vi "MainVI.vi"() -> ()   [LabVIEW 2022 SP3]
uses:
  <vilib>/Simulation/Scripting/Companion Diagram/SimConfigNode/SimParams.ctl
  <vilib>/Simulation/Scripting/Companion Diagram/SimConfigNode/_simSolvers.ctl
  <vilib>/Simulation/Implementation/Shared/SIMSCR Execution Mode.ctl
  <vilib>/Simulation/Param Hierarchy/Typedefs/SIMPH Param Control Actions.ctl
  <vilib>/OPCUA/controls/NodeId.ctl
  <vilib>/OPCUA/controls/Write Status.ctl
  <vilib>/Simulation/Implementation/Shared/NILVSim_ParamChanged.vi
  <vilib>/Simulation/Implementation/Shared/NILVSIM_BeginStep.vi
  <vilib>/Simulation/Implementation/Shared/NILVSim_Manager.vi
  <vilib>/Utility/error.llb/Clear Errors.vi
  <vilib>/Simulation/Implementation/Shared/NILVSim_FinalizeModel.vi
  <vilib>/Simulation/Implementation/Shared/SIM Unbundle Sim Info.vi
  <vilib>/Simulation/Implementation/Shared/NILVSim_Initialize.vi
  <vilib>/Simulation/Utility/Implementation/NILVSim Get Time and IsAcceptedStep.vi
  <vilib>/Simulation/Implementation/Shared/SIMSH Read Queue.vi
  <vilib>/Simulation/Implementation/Shared/NILVSim_GetModelError.vi
  <vilib>/Simulation/Implementation/Shared/SIM Bundle Sim Info.vi
  <vilib>/OPCUA/client/Multiple Write Double.vi
  <vilib>/Simulation/Implementation/XNodeFramework/SimXNode/SimX.xnode
  SubVI/Mathematical Model Air Heater.vi
  <vilib>/Simulation/Scripting/Companion Diagram/SimConfigNode/SimDog.xnode
  <vilib>/Simulation/Implementation/Shared/NI_SIM_Implementation.lvlib
  <vilib>/OPCUA/NI OPC UA Client.lvlib
panel:
  out "T_env [Deg C]":dbl caption="Environment \nTemperature [Deg C]" format="%.1g"
  out "Temperature Chart":T1(graph)
  out "Control Signal [V]":dbl(slide)=1.1413304392579737 scale=0.0..5.0
  in  "Tab Control":enum32{"Process", "Controller"}(tab)=enum."Controller"
  in  "Simulation":bool=TRUE
  in  "Model Parameters":T2={"K [C/V]"=3.5, "T_delay [s]"=2.0, "T_env [Deg C]"=21.5, "T initial [Deg C]"=21.5, "T [s]"=22.0}
  in  "PI Controller":bool=TRUE caption="Controller"
  in  "Manual Control [V]":dbl(slide) scale=0.0..5.0
  in  "PI Parameters":cluster{"Kp":dbl, "Ti [s]":dbl}={"Kp"=0.8, "Ti [s]"=20.0}
  in  "Control Signal Range":cluster{"u_max":dbl, "u_min":dbl}={"u_max"=5.0, "u_min"=0.0}
  out "Name":string
  in  "Setpoint [Deg C]":dbl=30.0
  in  "Ts [s]":dbl=0.1
  in  "Stop Button":bool
  out "Temperature [Deg C]":dbl(slide)=21.64553529889341 scale=20.0..50.0
  out "Error out":errorcluster
  in  "Error in":errorcluster
  # "Control Module"
  # "Simulation"
  # "Real"
  # "PI Controller"
  # "Manual Controller"
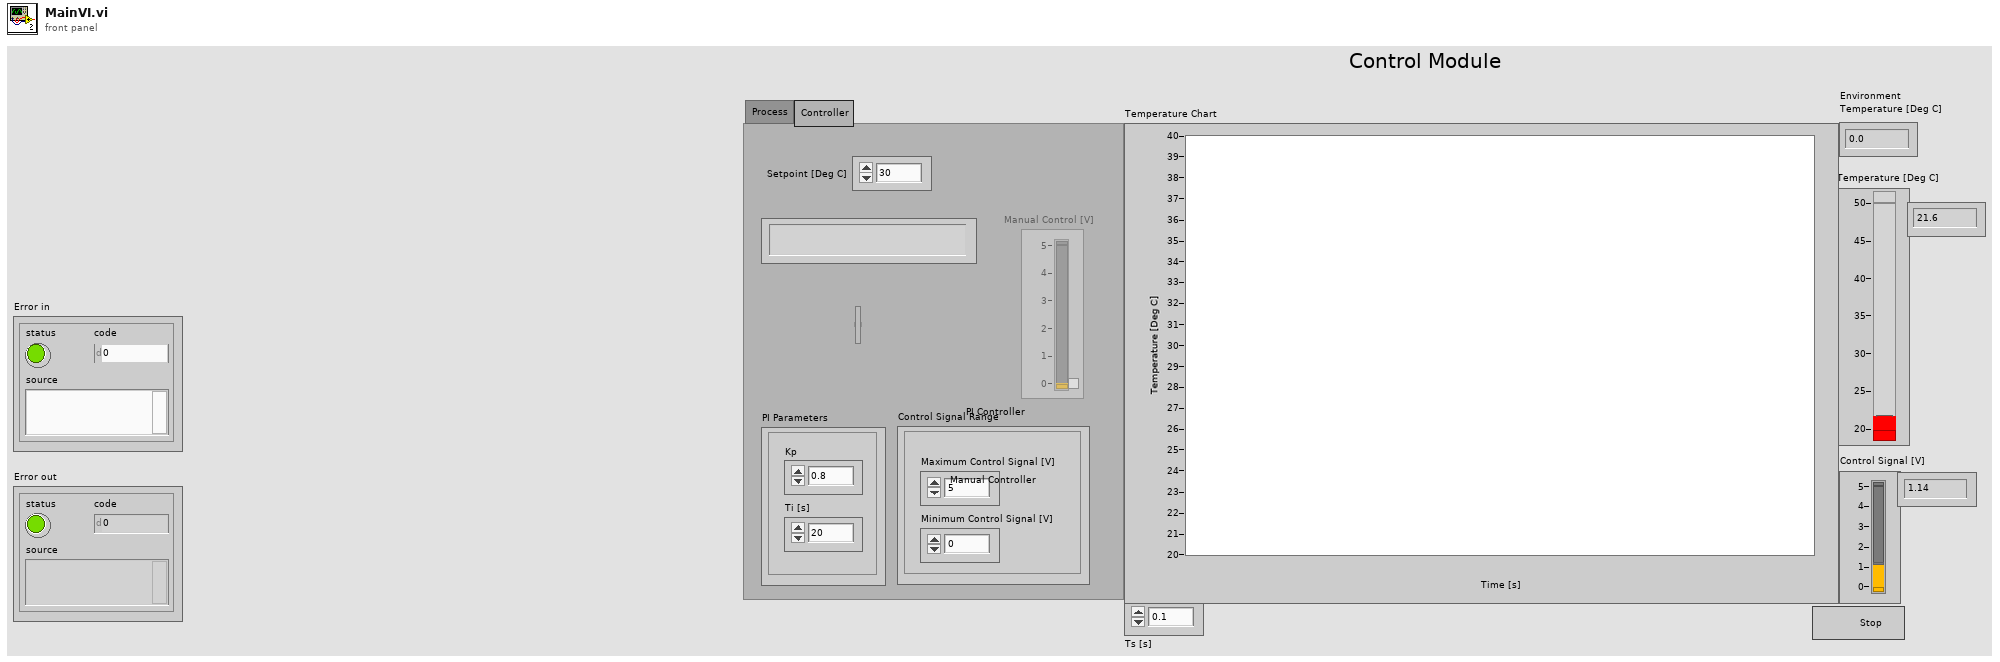
[diagram p1: front panel]
types:
  T1 = cluster{"T_out [deg C]":dbl, "Setpoint [Deg C]":dbl}
  T2 = cluster{"K [C/V]":dbl, "T_delay [s]":dbl, "T_env [Deg C]":dbl, "T initial [Deg C]":dbl, "T [s]":dbl}
  T3 = cluster{"T_out [deg C]":dbl, "Setpoint [Deg C]":dbl}[]
  T4 = enum8{"Enabled", "Disabled", "Disabled and Grayed Out"}
  T5 = enum16{"Simulate to Completion", "Single Time-Step Simulation (Fixed Step Only)"}
  T6 = typedef "SIMSCR Execution Mode.ctl" = enum16{"Simulate to Completion", "Single Time-Step Simulation (Fixed Step Only)"}
  T7 = typedef "SIMPH Param Control Actions.ctl" = enum16{"get params", "set params"}
  T8 = cluster{"SIMSH Sim Time":dbl, "Unbundle By Name":cluster{"K [C/V]":dbl, "T_delay [s]":dbl, "T_env [Deg C]":dbl, "T initial [Deg C]":dbl, "T [s]":dbl}, "Model Parameters":cluster{"K [C/V]":dbl, "T_delay [s]":dbl, "T_env [Deg C]":dbl, "T initial [Deg C]":dbl, "T [s]":dbl}, "Integrator":cluster{"output":dbl}, "Devision":cluster{"Result":dbl}, "Minus":cluster{"Result":dbl}, "Transport Delay":cluster{"output":dbl}, "Summation":cluster{"Result":dbl}, "Multiplication":cluster{"Result":dbl}}
  T9 = typedef "SimParams.ctl" = cluster{"Initial Time (s)":dbl, "Final Time (s)":dbl, "Step Size (s)":dbl, "ODE Solver":T10, "Minimum Step Size (s)":dbl, "Maximum Step Size (s)":dbl, "Relative Tolerance":dbl, "Absolute Tolerance":dbl, "Software Timing":bool, "Initial Step Size (s)":dbl, "Automatic Fixed Step Size?":bool, "Automatic Discrete Step Size?":bool, "Discrete Step Size (s)":dbl, "Calculate using Time Step":bool, "Solver Wired?":bool, "Prev.Frm.Expected End":u64, "Prev.Frm.Actual End":u64, "Prev.Frm.Finished Late?":bool, "Prev.Iter.Expected End":u64, "Prev.Iter.Actual End":u64, "Prev.Iter.Finished Late?":bool, "Expected Iteration Start":u64, "Actual Iteration Start":u64, "Expected Frame Start":u64, "Actual Frame Start":u64, "Source Name":string, "Name":string, "Period":i64, "Deadline":i64, "Offset":i64, "Start":i64, "Priority":i32, "Timeout":i32, "Processor":i32, "Mode":enum32{"No Change", "Process missed periods, maintain original phase", "Discard missed periods, maintain original phase", "Process missed periods, ignore original phase", "Discard missed periods, ignore original phase"}, "Wakeup reason":enum32{"Normal", "Aborted", "Asynchronous wakeup", "Timing source error", "Timed loop error", "Timeout"}, "Error":errorcluster, "Source Type":string, "Secondary Source Type":string, "Global End Time":u64, "Global Start Time":u64, "Full Solver Reset":bool, "Execution Mode":T6, "Nan/Inf Check":bool, "Custom Solver Library":string, "Solver Is Variable":bool, "custom solver name":string, "Signal Collection Decimation":u32}
  T10 = typedef "_simSolvers.ctl" = enum16{"Runge-Kutta 1 (Euler)", "Runge-Kutta 2", "Runge-Kutta 3", "Runge-Kutta 4", "Runge-Kutta 23 (variable)", "Runge-Kutta 45 (variable)", "BDF (variable)", "Adams-Moulton (variable)", "Rosenbrock (variable)", "Discrete States Only", "SDIRK 4 (variable)", "Radau 5 (variable)", "Radau 9 (variable)", "Radau 13 (variable)", "Radau [Variable Order] (variable)", "Gear's Method (variable)", "Linearizer", "State Query", "Trim Eval", "Custom Solver"}
  T11 = typedef "NodeId.ctl" = string
  T12 = cluster{"message mode":enum16{"None", "Sign", "Sign and Encrypt"}, "security":enum16{"Basic256", "Basic128Rsa15"}}
  T13 = typedef "OPC UA Client Refnum.ctl" = refnum<k21>
  T14 = cluster{"Filter Output":dbl, "Setpoint [Deg C]":dbl}
  T15 = cluster{"Setpoint [Deg C]":dbl, "Temperature [Deg C]":dbl}
  T16 = typedef "Write Status.ctl" = u32
  T17 = cluster{"node ID":T11, "value":dbl, "timestamp (current time)":timestamp, "node status":T16}
  T18 = cluster{"node ID":T11, "value":dbl, "timestamp (current time)":timestamp, "node status":T16}[]
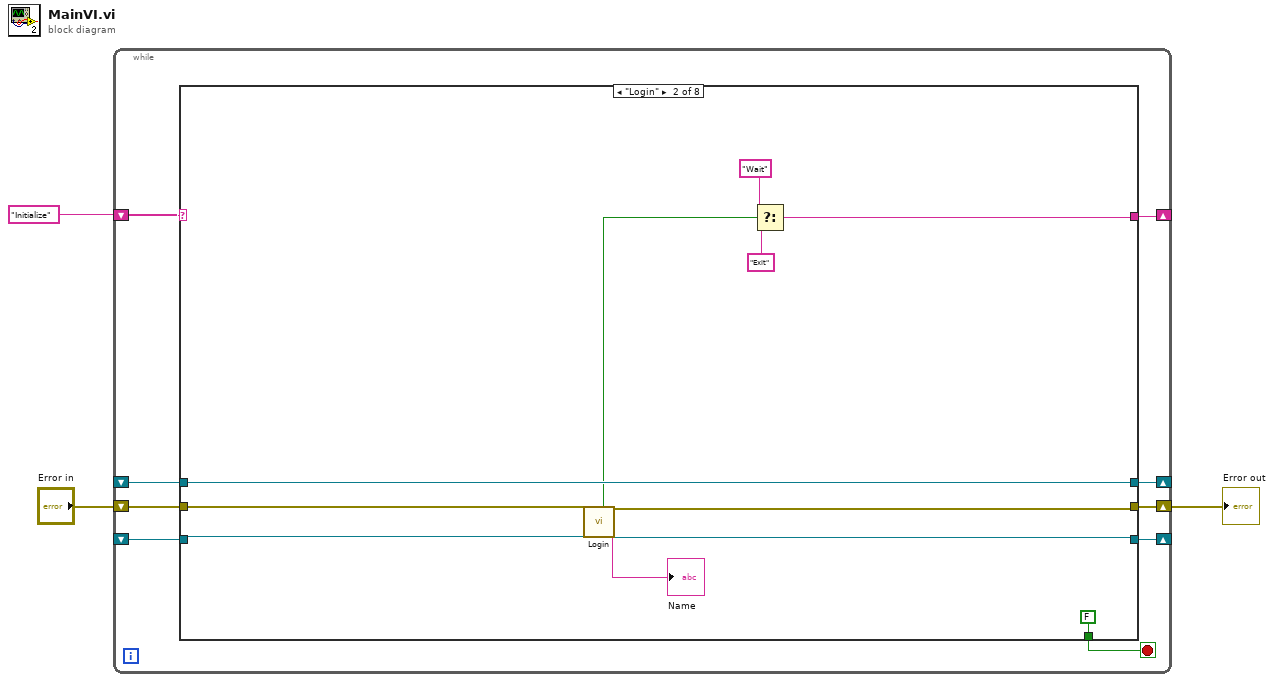
[diagram p0: block diagram]
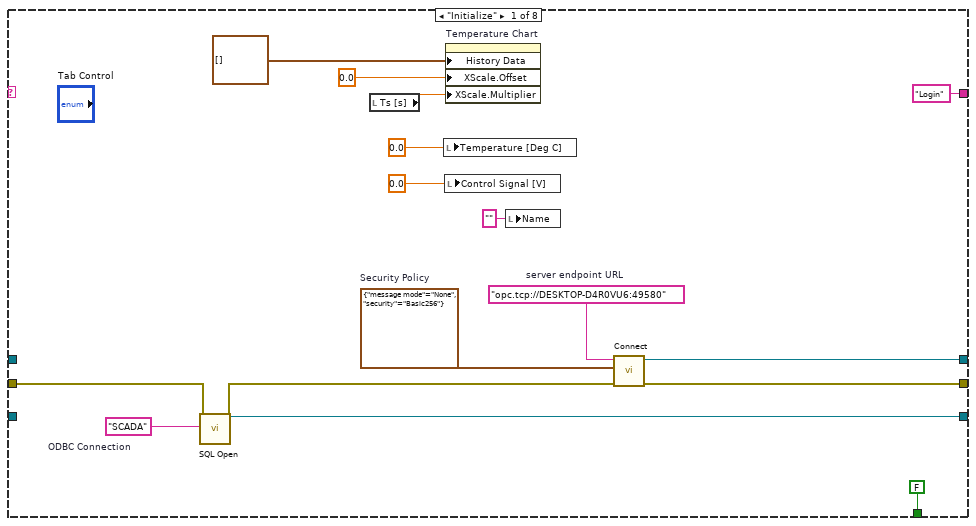
[diagram p2: hidden frame]
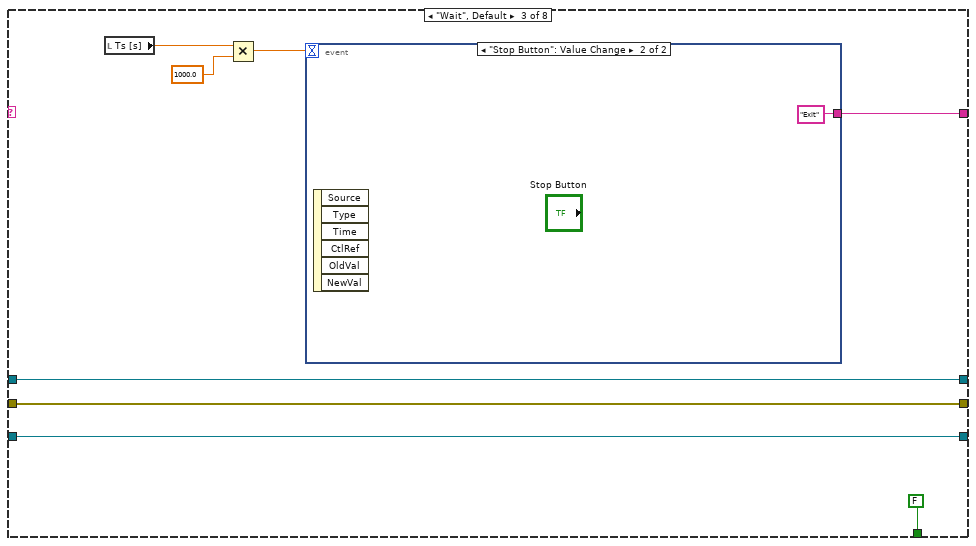
[diagram p3: hidden frame]
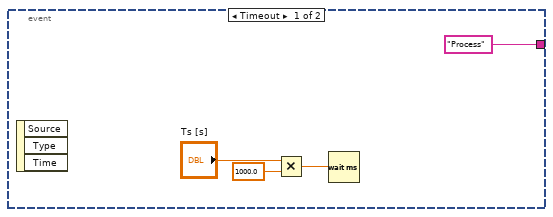
[diagram p4: hidden frame]
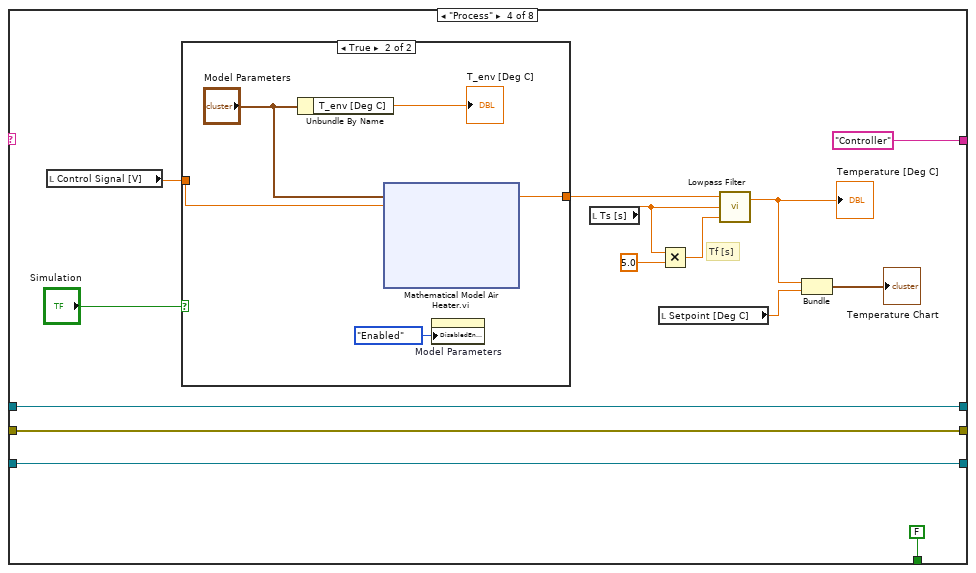
[diagram p5: hidden frame]
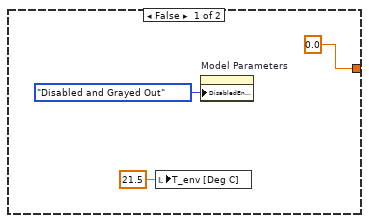
[diagram p6: hidden frame]
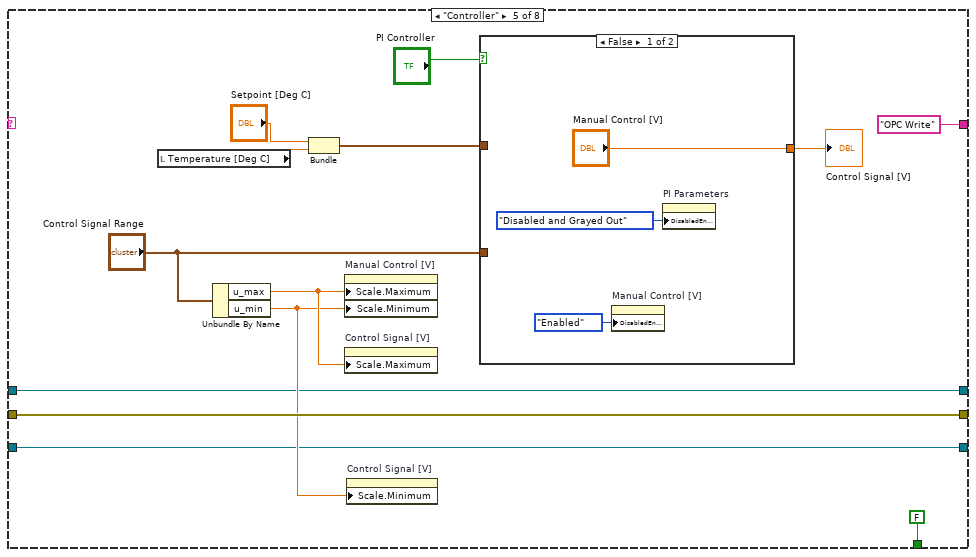
[diagram p7: hidden frame]
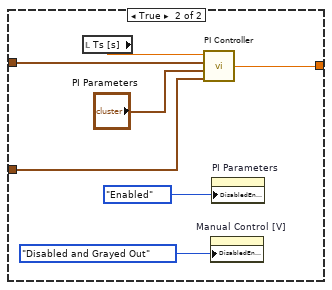
[diagram p8: hidden frame]
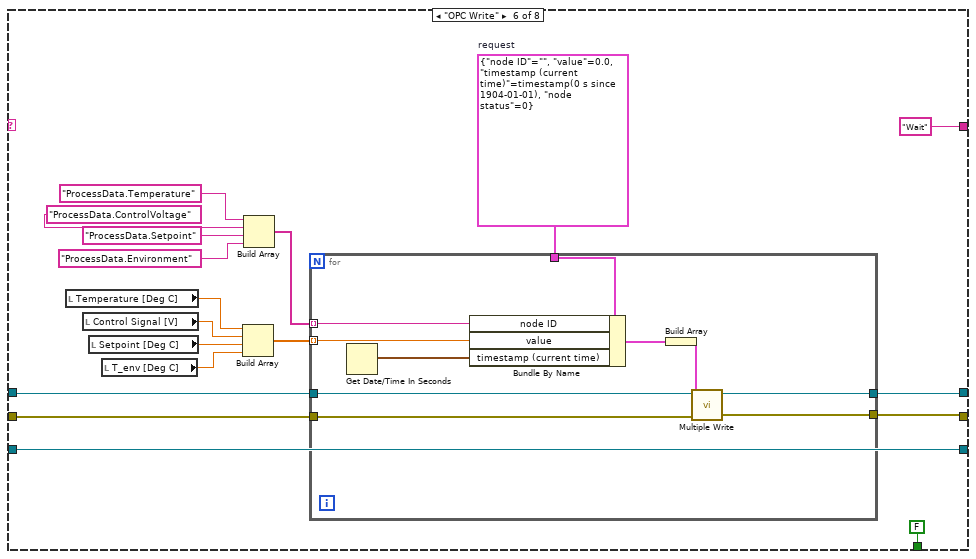
[diagram p9: hidden frame]
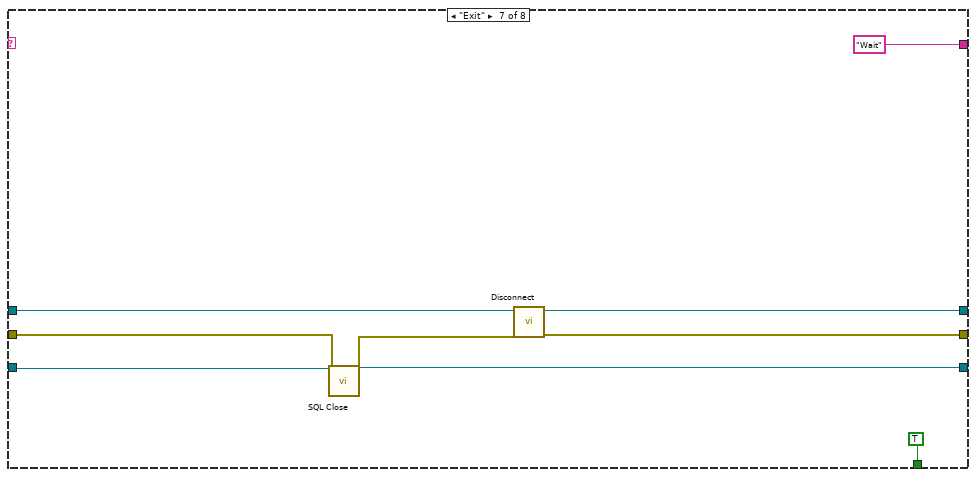
[diagram p10: hidden frame]
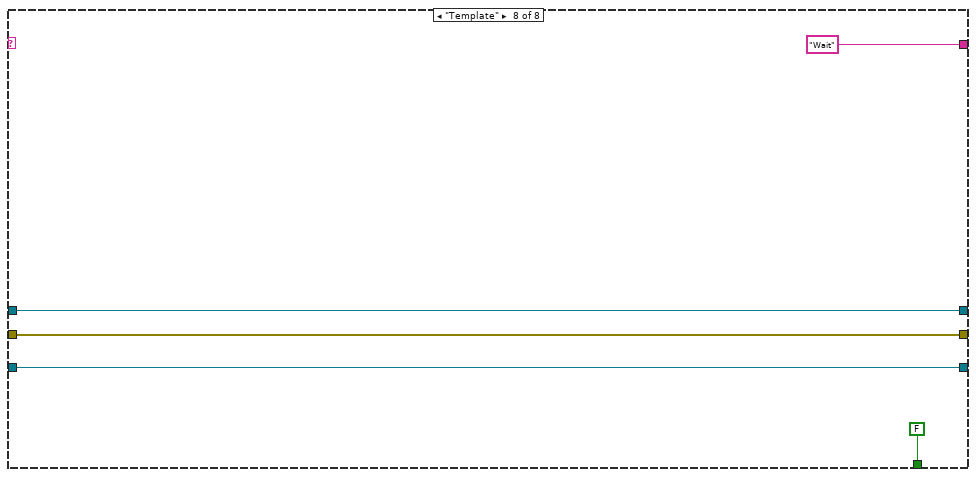
[diagram p11: hidden frame]
diagram:
  n1 = while {
    shift-right: [w11] -> _
    shift-left: "Initialize" -> [w12]
    shift-right: [w8] -> w1
    shift-left: "Error in" -> [w9]
    shift-right: [w7] -> _
    shift-left: _ -> [w6]
    shift-right: [w5] -> _
    shift-left: _ -> [w4]
    stop <- w10 stop-if-true
    n2 = case shown="\"Login\"" w12 {
      tunnel: ["Login" ("f") w34 w46 "Controller" "OPC Write" "Wait" "Wait" "Wait"] -> w11
      tunnel: [FALSE FALSE FALSE FALSE FALSE FALSE TRUE FALSE] -> w10
      tunnel: w9 -> [w17 w32 w42 w62 w333 w355 w378 w386]
      tunnel: [w21 w31 w42 w62 w333 w354 w381 w386] -> w8
      tunnel: [w19 w39 w41 w54 w327 w352 w380 w385] -> w7
      tunnel: w6 -> [_ w39 w41 w54 w327 w353 w380 w385]
      tunnel: [w15 w29 w40 w53 w326 w349 w379 w384] -> w5
      tunnel: w4 -> [_ w30 w40 w53 w326 w349 w379 w384]
      frame "Initialize" {
        w18 = "SCADA"  # ODBC Connection
        w22 = T12 {"message mode"=enum."None", "security"=enum."Basic256"}  # Security Policy
        w23 = "opc.tcp://DESKTOP-D4R0VU6:49580"  # server endpoint URL
        n3 = call <vilib>:"SQL Open.vi"("ConnectionString In"=w18, "Error in (no error)"=w17) -> ("Connection Out"=w15:refnum<k7>, "Error out"=w16:errorcluster)  [unwired: 16 in]
        n4 = local read "Ts [s]"() -> (w25:dbl)
        n5 = local write "Temperature [Deg C]"(0.0 ("Thermometer")) -> ()
        n6 = local write "Control Signal [V]"(0.0 ("Control Signal [V]")) -> ()
        n7 = property on="Temperature Chart" class="WFChart (strict)"("History Data"=T3 [], "XScale.Offset"=0.0 ("X Scale.Offset and Multiplier:Offset"), "XScale.Multiplier"=w25) -> ()  [unwired: 2 in, 2 out]
        n8 = local write "Name"("" ("Name")) -> ()
        n9 = call <vilib>:"Connect.vi"("error in (no error)"=w16, "security policy"=w22, "server endpoint URL"=w23) -> ("error out"=w21:errorcluster, "OPC UA client refnum out"=w19:T13)  [unwired: 6 in, 1 out]
      }
      frame "Login" {
        n10 = call "Login.vi"("Connection In"=w30, "error in"=w32) -> ("Not empty?"=w37:bool, "error out"=w31:errorcluster, "Connection Out"=w29:refnum<k7>, "Name"=→"Name":string)  [unwired: 2 out]
        n11 = Select(t="Wait", s=w37, f="Exit") -> (s? t:f=w34:string)
      }
      frame "Wait", Default {
        n12 = local read "Ts [s]"() -> (w45:dbl)
        n13 = Multiply(x=w45, y=1000.0) -> (x*y=w43:dbl)
        n14 = event shown="[1] \"Stop Button\": Value Change" {
          selector: _ -> [_ _]
          dyn-events: _ -> [_ _]
          timeout: w43 -> [_ _]
          tunnel: ["Process" "Exit"] -> w46
          event Timeout {
            n15 = event-data() -> ()  [unwired: 1 in, 3 out]
            n16 = Multiply(x="Ts [s]", y=1000.0) -> (x*y=w48:dbl)
            n17 = Wait (ms)(milliseconds to wait=w48) -> ()  [unwired: 1 out]
          }
          event "Stop Button": Value Change {
            n18 = event-data() -> ()  [unwired: 1 in, 6 out]
          }
        }
      }
      frame "Process" {
        # "Tf [s]"
        n19 = local read "Control Signal [V]"() -> (w63:dbl)
        n20 = case shown="True" "Simulation" {
          tunnel: [0.0 ("T_out [deg C]") w74] -> w58
          tunnel: w63 -> [_ w73]
          frame False {
            n21 = local write "T_env [Deg C]"(21.5 ("T_env [Deg C]")) -> ()
            n22 = property on="Model Parameters" class="Clust (strict)"("DisabledEnum"=T4."Disabled and Grayed Out" ("Disabled")) -> ()  [unwired: 2 in, 2 out]
          }
          frame True {
            n23 = Unbundle By Name("Model Parameters") -> ("T_env [Deg C]"=→"T_env [Deg C]":dbl)
            n24 = xnode "Mathematical Model Air Heater.vi"("Model Parameters"="Model Parameters", "u [V]"=w73) -> ("T_out [deg C]"=w74:dbl)  [unwired: 2 in, 1 out]
            n25 = property on="Model Parameters" class="Clust (strict)"("DisabledEnum"=T4."Enabled" ("Disabled")) -> ()  [unwired: 2 in, 2 out]
          }
        }
        n26 = local read "Ts [s]"() -> (w57:dbl)
        n27 = local read "Setpoint [Deg C]"() -> (w61:dbl)
        n28 = Multiply(x=w57, y=5.0) -> (x*y=w55:dbl)
        n29 = call "Lowpass Filter.vi"("Tf [s]"=w55, "Ts [s]"=w57, "Fillter input"=w58) -> ("Filter Output"=w59:dbl)  [unwired: 1 in]
        "Temperature [Deg C]" <- w59
        n30 = Bundle "Bundle"("Filter Output"=w59, "Setpoint [Deg C]"=w61) -> (→"Temperature Chart":T14)  [unwired: 1 in]
      }
      frame "Controller" {
        n31 = local read "Temperature [Deg C]"() -> (w331:dbl)
        n32 = Unbundle By Name "Unbundle By Name"("Control Signal Range") -> ("u_max"=w329:dbl, "u_min"=w328:dbl)
        n33 = Bundle("Setpoint [Deg C]"="Setpoint [Deg C]", "Temperature [Deg C]"=w331) -> (w330:T15)  [unwired: 1 in]
        n34 = property on="Manual Control [V]" class="Slide (strict)"("Scale.Maximum"=w329, "Scale.Minimum"=w328) -> ()  [unwired: 2 in, 2 out]
        n35 = property on="Control Signal [V]" class="Slide (strict)"("Scale.Maximum"=w329) -> ()  [unwired: 2 in, 2 out]
        n36 = property on="Control Signal [V]" class="Slide (strict)"("Scale.Minimum"=w328) -> ()  [unwired: 2 in, 2 out]
        n37 = case shown="False" "PI Controller" {
          tunnel: ["Manual Control [V]" w345] -> w336
          tunnel: "Control Signal Range" -> [_ w344]
          tunnel: w330 -> [_ w343]
          frame False {
            n38 = property on="Manual Control [V]" class="Slide (strict)"("DisabledEnum"=T4."Enabled" ("Disabled")) -> ()  [unwired: 2 in, 2 out]
            n39 = property on="PI Parameters" class="Clust (strict)"("DisabledEnum"=T4."Disabled and Grayed Out" ("Disabled")) -> ()  [unwired: 2 in, 2 out]
          }
          frame True {
            n40 = local read "Ts [s]"() -> (w347:dbl)
            n41 = call "PI Controller.vi"("Control Signal Range"=w344, "PI Parameters"="PI Parameters", "Process"=w343, "Ts [s]"=w347) -> ("Output"=w345:dbl)
            n42 = property on="Manual Control [V]" class="Slide (strict)"("DisabledEnum"=T4."Disabled and Grayed Out" ("Disabled")) -> ()  [unwired: 2 in, 2 out]
            n43 = property on="PI Parameters" class="Clust (strict)"("DisabledEnum"=T4."Enabled" ("Disabled")) -> ()  [unwired: 2 in, 2 out]
          }
        }
        "Control Signal [V]" <- w336
      }
      frame "OPC Write" {
        w364 = T17 {"node ID"="", "value"=0.0, "timestamp (current time)"=timestamp(0 s since 1904-01-01), "node status"=0}  # request
        n44 = local read "Temperature [Deg C]"() -> (w361:dbl)
        n45 = local read "Control Signal [V]"() -> (w358:dbl)
        n46 = local read "Setpoint [Deg C]"() -> (w359:dbl)
        n47 = local read "T_env [Deg C]"() -> (w351:dbl)
        n48 = Build Array(w361, w358, w359, w351) -> (w360:dbl[])
        n49 = Build Array(T11 "ProcessData.Temperature" ("node ID"), T11 "ProcessData.ControlVoltage" ("node ID"), T11 "ProcessData.Setpoint" ("node ID"), T11 "ProcessData.Environment" ("element")) -> (w362:T11[])
        n50 = for {
          tunnel: w364 -> [w376]
          tunnel: w362 -> [w375] mode=indexing
          tunnel: w360 -> [w374] mode=indexing
          tunnel: w355 -> [w371]
          tunnel: [w370] -> w354
          tunnel: w353 -> [w368]
          tunnel: [w367] -> w352
          n51 = Get Date/Time In Seconds() -> (seconds since 1Jan1904=w369:timestamp)
          n52 = Bundle By Name "Bundle By Name"(cluster=w376, "node ID"=w375, "value"=w374, "timestamp (current time)"=w369) -> (w373:T17)
          n53 = Build Array "Build Array"(w373) -> (w372:T18)
          n54 = call-poly <vilib>:"Multiple Write.vi"("error in (no error)"=w371, "requests"=w372, "OPC UA client refnum in"=w368) -> ("error out"=w370:errorcluster, "OPC UA client refnum out"=w367:T13)  [unwired: 5 in, 2 out]
        }
      }
      frame "Exit" {
        n55 = call <vilib>:"SQL Close.vi"("Connection In"=w379, "Error in (no error)"=w378) -> ("Error out"=w377:errorcluster)  [unwired: 17 in]
        n56 = call <vilib>:"Disconnect.vi"("error in (no error)"=w377, "OPC UA client refnum in"=w380) -> ("error out"=w381:errorcluster)  [unwired: 9 in]
      }
      frame "Template" {
      }
    }
  }
  "Error out" <- w1
